vi "Add.vi"(8 "error in (no error)":errorcluster, 10 "Data2D 2":refnum<class "Data2D.lvclass">, 11 "Data2D in":refnum<class "Data2D.lvclass">) -> (0 "error out":errorcluster, 3 "Data2D out":refnum<class "Data2D.lvclass">)   [LabVIEW 2014, in "Data2D.lvclass"]
uses:
  Data2D.lvclass
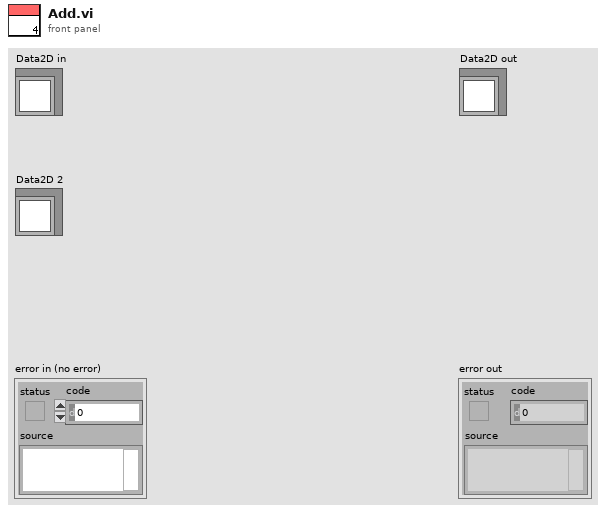
[diagram p1: front panel]
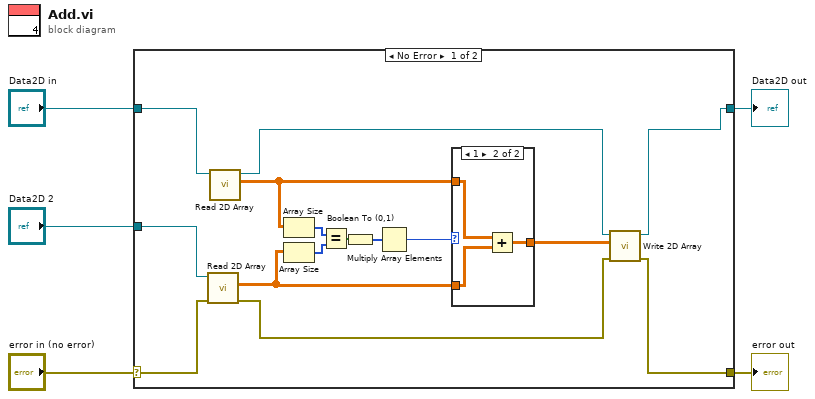
[diagram p0: block diagram]
diagram:
  n1 = case shown="No Error" "error in (no error)" {
    selector: "error in (no error)" -> [w13 w26]
    tunnel: [w15 w26] -> w4
    tunnel: [w16 w25] -> w2
    tunnel: "Data2D in" -> [w19 w25]
    tunnel: "Data2D 2" -> [w14 _]
    frame No Error {
      n2 = call "Read 2D Array.vi"("error in (no error)"=w13, "Data2D in"=w14) -> ("error out"=w11:errorcluster, "2D Array"=w12:dbl[][])  [unwired: 7 in, 1 out]
      n3 = call "Read 2D Array.vi"("Data2D in"=w19) -> ("2D Array"=w18:dbl[][], "Data2D out"=w17:refnum<class "Data2D.lvclass">)  [unwired: 8 in, 1 out]
      n4 = Array Size(array=w18) -> (size(s)=w9:i32[])
      n5 = Array Size(array=w12) -> (size(s)=w20:i32[])
      n6 = Equal?(x=w9, y=w20) -> (x = y?=w8:bool[])
      n7 = Boolean To (0,1)(Boolean=w8) -> (0, 1=w7:i16[])
      n8 = Multiply Array Elements(1:w7) -> (0:w6:i16)
      n9 = case shown="1" w6 {
        tunnel: w18 -> [_ w24]
        tunnel: w12 -> [w21 w23]
        tunnel: [w21 w22] -> w10
        frame 0, Default {
        }
        frame 1 {
          n10 = Add(x=w24, y=w23) -> (x+y=w22:dbl[][])
        }
      }
      n11 = call "Write 2D Array.vi"("error in (no error)"=w11, "2D Array"=w10, "Data2D in"=w17) -> ("error out"=w15:errorcluster, "Data2D out"=w16:refnum<class "Data2D.lvclass">)  [unwired: 7 in]
    }
    frame Error {
    }
  }
  "error out" <- w4
  "Data2D out" <- w2
